vi "Position_InsideTab.vi"(6 "Extra":dbl format="%#_13g", 7 "Top":dbl=5.0 format="%#_13g", 8 "error in (no error)":errorcluster, 10 "FirstLineSettings":refnum<vi>[](array[refnum]), 11 "TabControl in":refnum<vi>) -> (0 "error out":errorcluster, 1 "Width":dbl, 2 "Left":dbl, 3 "Top":dbl)   [LabVIEW 2021]
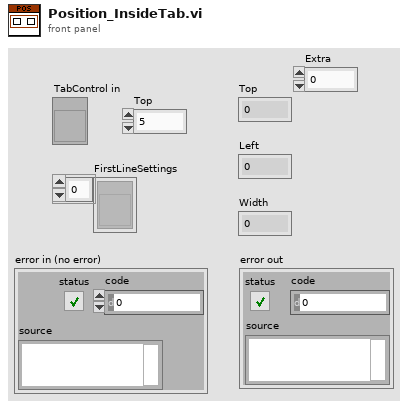
[diagram p1: front panel]
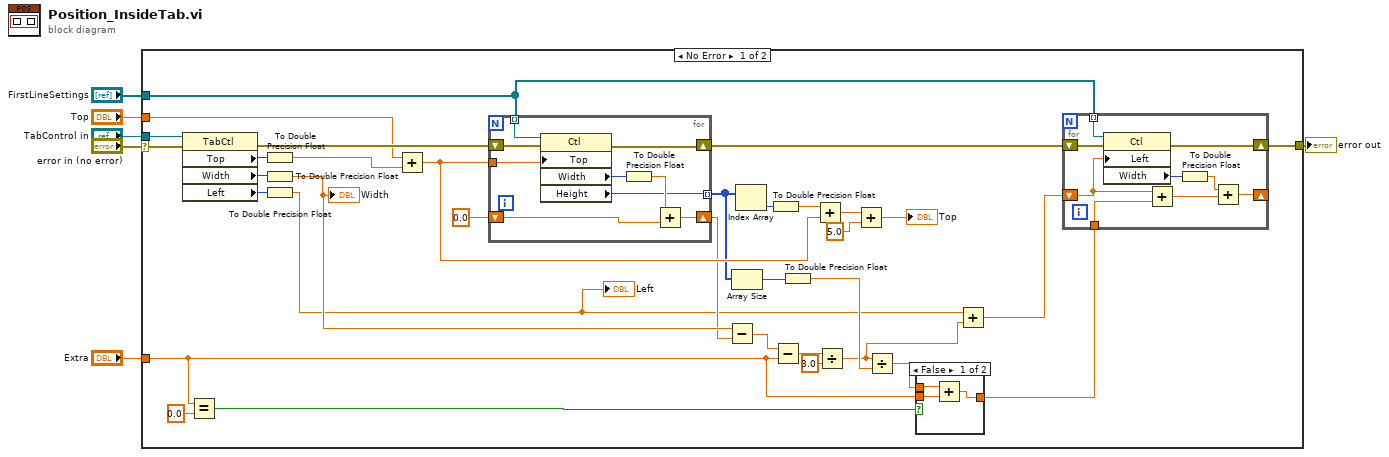
[diagram p0: block diagram]
diagram:
  n1 = case shown="No Error" "error in (no error)" {
    selector: "error in (no error)" -> [w40 w63]
    tunnel: [w39 w63] -> w5
    tunnel: "FirstLineSettings" -> [w29 _]
    tunnel: "TabControl in" -> [w24 _]
    tunnel: "Top" -> [w14 _]
    tunnel: "Extra" -> [w9 _]
    frame No Error {
      n2 = property on="Property Node" class="TabCtl"(reference=w24, error in=w40) -> (error out=w26:errorcluster, "Top"=w25:i32, "Width"=w27:u32, "Left"=w36:i32)  [unwired: 1 out]
      n3 = Equal?(x=w9, y=0.0) -> (x = y?=w20:bool)
      n4 = To Double Precision Float(number=w25) -> (double precision float=w15:dbl)
      n5 = To Double Precision Float(number=w27) -> (double precision float=w35:dbl)
      "Width" <- w35
      n6 = To Double Precision Float(number=w36) -> (double precision float=w8:dbl)
      "Left" <- w8
      n7 = Add(x=w14, y=w15) -> (x+y=w32:dbl)
      n8 = for {
        shift-right: [w57] -> w28
        shift-left: w26 -> [w62]
        tunnel: w29 -> [w61] mode=indexing
        tunnel: w32 -> [w60]
        shift-right: [w59] -> w19
        shift-left: 0.0 -> [w58]
        tunnel: [w54] -> w12 mode=indexing
        n9 = property class="Ctl"(reference=w61, error in=w62, "Top"=w60) -> (error out=w57:errorcluster, "Width"=w56:u32, "Height"=w54:u32)  [unwired: 1 out]
        n10 = To Double Precision Float(number=w56) -> (double precision float=w55:dbl)
        n11 = Add(x=w55, y=w58) -> (x+y=w59:dbl)
      }
      n12 = Subtract(x=w35, y=w19) -> (x-y=w18:dbl)
      n13 = Array Size(array=w12) -> (size(s)=w13:i32)
      n14 = Index Array(array=w12) -> (element=w31:u32)  [unwired: 1 in]
      n15 = To Double Precision Float(number=w31) -> (double precision float=w30:dbl)
      n16 = Subtract(x=w18, y=w9) -> (x-y=w17:dbl)
      n17 = To Double Precision Float(number=w13) -> (double precision float=w11:dbl)
      n18 = Add(x=w30, y=w32) -> (x+y=w33:dbl)
      n19 = Divide(x=w17, y=3.0) -> (x/y=w7:dbl)
      n20 = Add(x=w33, y=5.0) -> (x+y=→"Top":dbl)
      n21 = Divide(x=w7, y=w11) -> (x/y=w10:dbl)
      n22 = case shown="False" w20 {
        tunnel: [w43 w44] -> w21
        tunnel: w10 -> [w42 w44]
        tunnel: w9 -> [w41 _]
        frame False {
          n23 = Add(x=w42, y=w41) -> (x+y=w43:dbl)
        }
        frame True {
        }
      }
      n24 = Add(x=w8, y=w7) -> (x+y=w37:dbl)
      n25 = for {
        shift-right: [w49] -> w39
        shift-left: w28 -> [w53]
        tunnel: w29 -> [w52] mode=indexing
        tunnel: w21 -> [w51]
        shift-right: [w45] -> _
        shift-left: w37 -> [w50]
        n26 = property class="Ctl"(reference=w52, error in=w53, "Left"=w50) -> (error out=w49:errorcluster, "Width"=w47:u32)  [unwired: 1 out]
        n27 = Add(x=w50, y=w51) -> (x+y=w48:dbl)
        n28 = To Double Precision Float(number=w47) -> (double precision float=w46:dbl)
        n29 = Add(x=w46, y=w48) -> (x+y=w45:dbl)
      }
    }
    frame Error {
    }
  }
  "error out" <- w5
